vi "wait_for_value_change.vi"   [LabVIEW 2015]
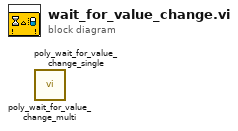
[diagram p0: block diagram]
diagram:
  n1 = call "poly_wait_for_value_change_multi.vi"() -> ()  [unwired: 10 in, 2 out]
  n2 = call "poly_wait_for_value_change_single.vi"() -> ()  [unwired: 10 in, 2 out]
